vi "Add BaseNodeType Child.vi"(8 "error in":errorcluster, 10 "child BaseNodeType in":refnum<k39>, 11 "parent ref in":T1 format="%.0x") -> (0 "error out":errorcluster, 1 "child ref":T1 format="%.0x", 2 "child BaseNodeType out":refnum<k39>, 3 "parent ref out":T1 format="%.0x")   [LabVIEW 2027, in "Custom Device Serialization.lvlib"]
uses:
  Custom Device Serialization.lvlib
  System Explorer Action.ctl
  C:/NetCoreDLL/NationalInstruments.VeriStand.SystemStorage.dll
  NetCoreDLL/NationalInstruments.VeriStand.SystemStorage.dll
  <vilib>/NI VeriStand/Custom Device API/Custom Device Item Ref.ctl
  <vilib>/NI VeriStand/Custom Device API/Custom Device API.lvlib
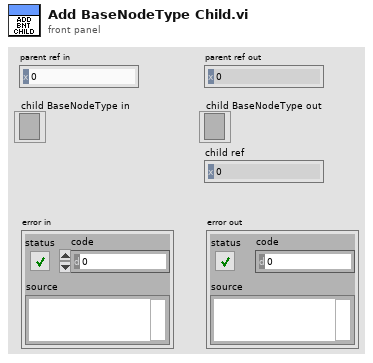
[diagram p1: front panel]
types:
  T1 = typedef "Custom Device API.lvlib/Custom Device Item Ref.ctl" = u64
  T2 = typedef "Custom Device Serialization.lvlib/System Explorer Action.ctl" = u16
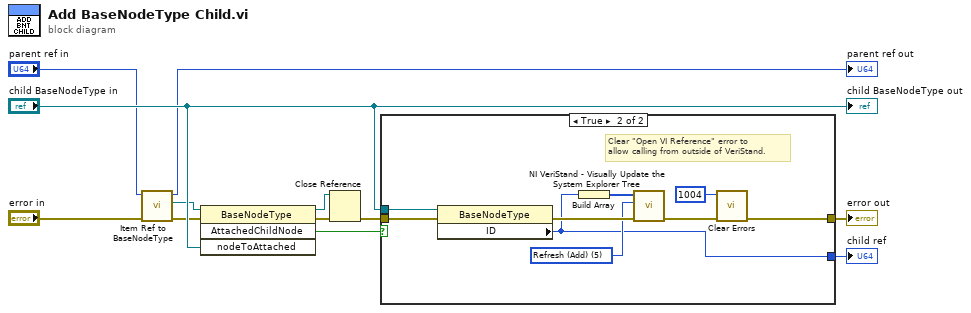
[diagram p0: block diagram]
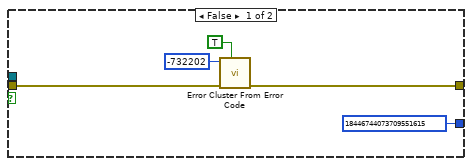
[diagram p2: hidden frame]
diagram:
  n1 = call "Item Ref to BaseNodeType.vi"("error in (no error)"="error in", "item ref in"="parent ref in") -> ("error out"=w11:errorcluster, "NationalInstruments.VeriStand.SystemStorage.BaseNodeType"=w9:refnum<k39>, "item ref out"=→"parent ref out":T1)  [unwired: 7 in]
  n2 = invoke class="BaseNodeType" method="AttachedChildNode"(reference=w9, error in=w11, "nodeToAttached"="child BaseNodeType in") -> (reference out=w5:refnum<k39>, error out=w6:errorcluster, "AttachedChildNode"=w1:bool)  [unwired: 1 in, 1 out]
  n3 = Close Reference(reference=w5, error in (no error)=w6) -> (error out=w8:errorcluster)
  n4 = case shown="True" w1 {
    tunnel: "child BaseNodeType in" -> [_ w26]
    tunnel: [w15 w23] -> w7
    tunnel: [u64 18446744073709551615 ("ID") w18] -> w2
    tunnel: w8 -> [w17 w24]
    frame False {
      n5 = call <vilib>:"Error Cluster From Error Code.vi"("show call chain? (False)"=TRUE, "error in (no error)"=w17, "error code (0)"=-732202) -> ("error out"=w15:errorcluster)  [unwired: 6 in]
    }
    frame True {
      w20 = T2 5 items=["Refresh (Add)"=5, "Refresh (Repopulate node)"=7, "Refresh (Delete)"=9] ("Action")
      # "Clear \"Open VI Reference\" error to\nallow calling from outside of VeriStand."
      n6 = property class="BaseNodeType"(reference=w26, error in=w24) -> (error out=w25:errorcluster, "ID"=w18:u64)  [unwired: 1 out]
      n7 = Build Array(w18) -> (w19:u64[])
      n8 = call "NI VeriStand - Visually Update the System Explorer Tree.vi"("error in (no error)"=w25, "Action"=w20, "Node IDs"=w19) -> ("error out"=w22:errorcluster)  [unwired: 8 in]
      n9 = call <vilib>:"Clear Errors.vi"("error in (no error)"=w22, "specific error code to clear (0: all)"=1004) -> ("error out"=w23:errorcluster)  [unwired: 4 in, 1 out]
    }
  }
  "error out" <- w7
  "child ref" <- w2
  "child BaseNodeType out" <- "child BaseNodeType in"
